vi "Auto-Pilot.vi"() -> ()   [LabVIEW 2017]
uses:
  <vilib>/Rock Robotics/WPI/DriverStation/WPI_DriverStationPositionInfo.ctl
  <vilib>/Rock Robotics/WPI/Utilities/WPI_GetSetVariantRefNum.vi
panel:
  out "Distance 6":dbl
  out "Distance 5":dbl
  out "Distance 2":dbl
  out "Distance":dbl
  out "substring":string
  out "Position":T1
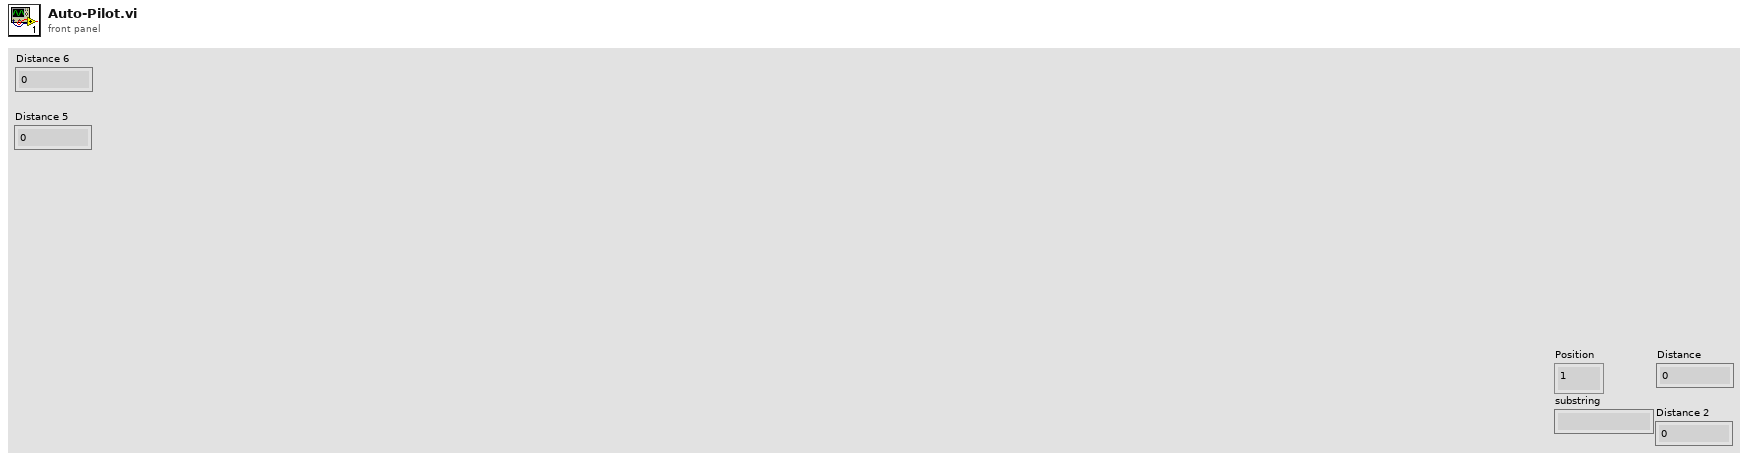
[diagram p1: front panel]
types:
  T1 = typedef "WPI_DriverStationPositionInfo.ctl" = enum16{"1", "2", "3"}
  T2 = typedef "WPI_EncoderDevRef.ctl" = cluster{"DevStatus":errorcluster, "EncoderIndex":T3, "CounterIndex":T4, "DistancePerCount":dbl, "Decoding Type":T5}
  T3 = typedef "FPGA_EncoderIdx.ctl" = enum8{"Enc 0", "Enc 1", "Enc 2", "Enc 3", "Enc 4", "Enc 5", "Enc 6", "Enc 7", "Invalid"}
  T4 = typedef "FPGA_CounterCtrSystemIndex.ctl" = enum8{"Ctr 0", "Ctr 1", "Ctr 2", "Ctr 3", "Ctr 4", "Ctr 5", "Ctr 6", "Ctr 7", "Invalid"}
  T5 = typedef "WPI_EncoderType.ctl" = enum16{"1x", "2x", "4x"}
  T6 = typedef "WPI_RobotDriveDevRef.ctl" = cluster{"DevStatus":errorcluster, "Motors[]":T7[], "Square Inputs":bool, "Max Output":dbl}
  T7 = typedef "WPI_MotorControlDeviceRef.ctl" = cluster{"DeviceStatus":errorcluster, "Type":T8, "PWM":cluster{"PWM Channel":T9, "DeadBand":T10}, "CAN":cluster{"Device Number":u8, "SetOutput VI Ref":variant, "GetOutput VI Ref":variant, "Enable VI Ref":variant, "Disable VI Ref":variant, "Data":variant}, "Invert":bool, "DIO PWM":cluster{"PWM \"Enable\" Channel":T9, "DIOChannel":T11, "PWM Rate":dbl}}
  T8 = typedef "WPI_MotorControlType.ctl" = enum16{"PWM", "CAN", "DIO PWM"}
  T9 = typedef "FPGA_DIOPWMChannel.ctl" = enum8{"PWM 0", "PWM 1", "PWM 2", "PWM 3", "PWM 4", "PWM 5", "PWM 6", "PWM 7", "PWM 8", "PWM 9", "PWM MXP 0", "PWM MXP 1", "PWM MXP 2", "PWM MXP 3", "PWM MXP 4", "PWM MXP 5", "PWM MXP 6", "PWM MXP 7", "PWM MXP 8", "PWM MXP 9", "Invalid"}
  T10 = typedef "WPI_PWMDeadband.ctl" = cluster{"Name":string, "maxPositivePwm":i32, "minPositivePwm":i32, "centerPwm":i32, "maxNegativePwm":i32, "minNegativePwm":i32, "angularRange":u16}
  T11 = typedef "FPGA_DIOChannel.ctl" = enum8{"DIO 0", "DIO 1", "DIO 2", "DIO 3", "DIO 4", "DIO 5", "DIO 6", "DIO 7", "DIO 8", "DIO 9", "DIO MXP 0", "DIO MXP 1", "DIO MXP 2", "DIO MXP 3", "DIO MXP 4", "DIO MXP 5", "DIO MXP 6", "DIO MXP 7", "DIO MXP 8", "DIO MXP 9", "DIO MXP 10", "DIO MXP 11", "DIO MXP 12", "DIO MXP 13", "DIO MXP 14", "DIO MXP 15", "SPI Port CS1", "SPI Port CS2", "SPI Port CS3", "SPI Port MISO", "SPI Port MOSI", "Invalid"}
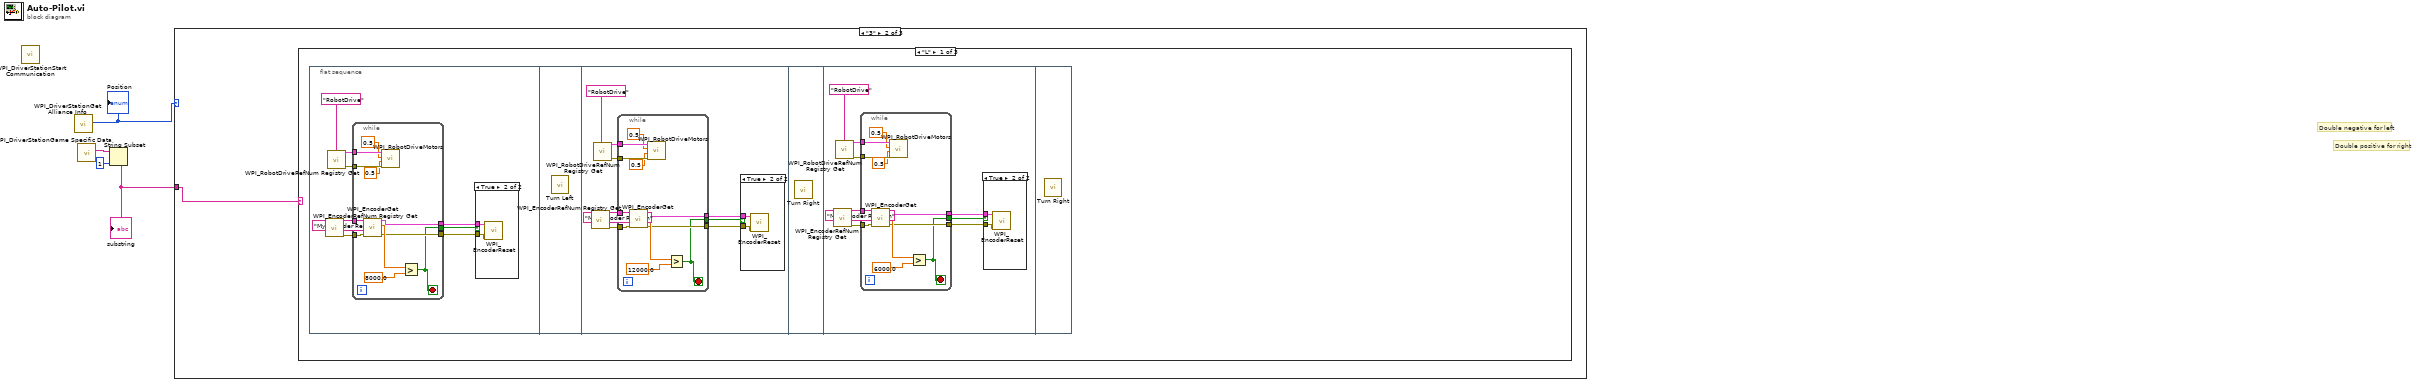
[diagram p0: block diagram]
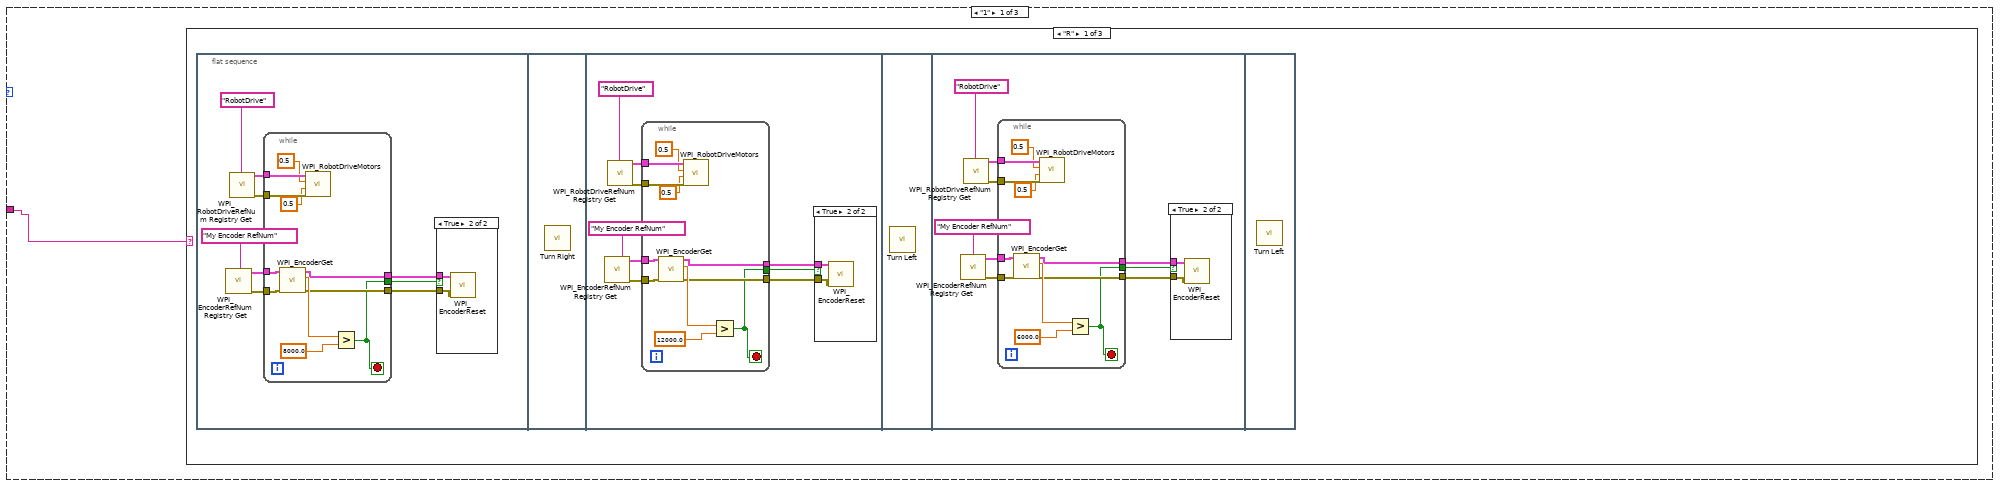
[diagram p2: hidden frame]
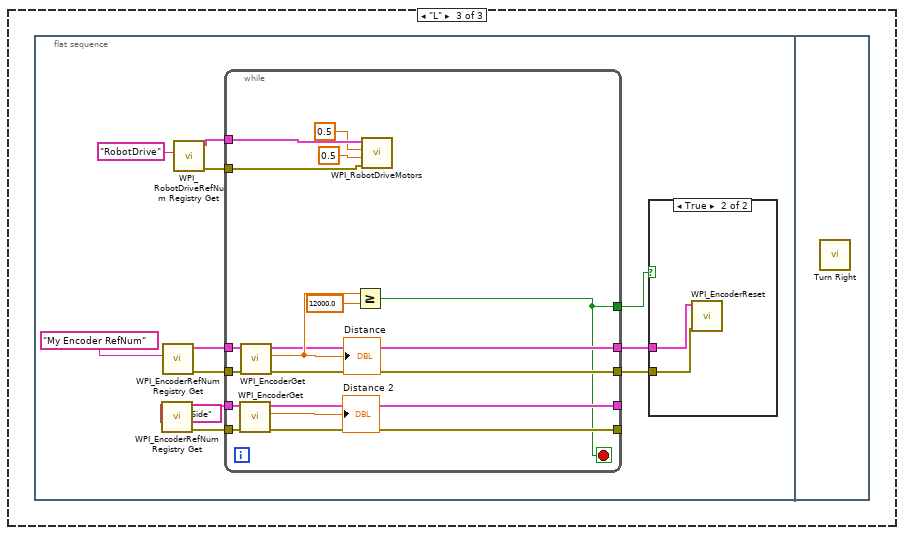
[diagram p7: hidden frame]
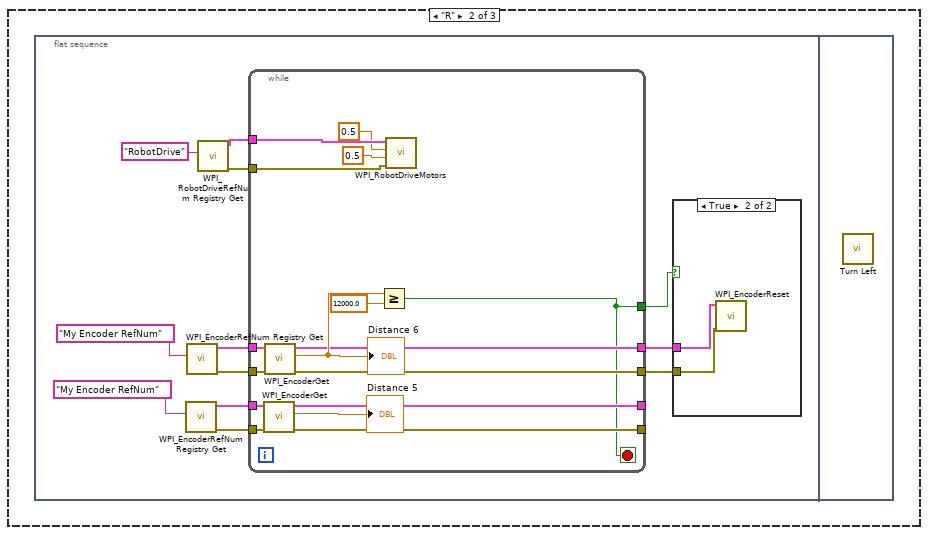
[diagram p12: hidden frame]
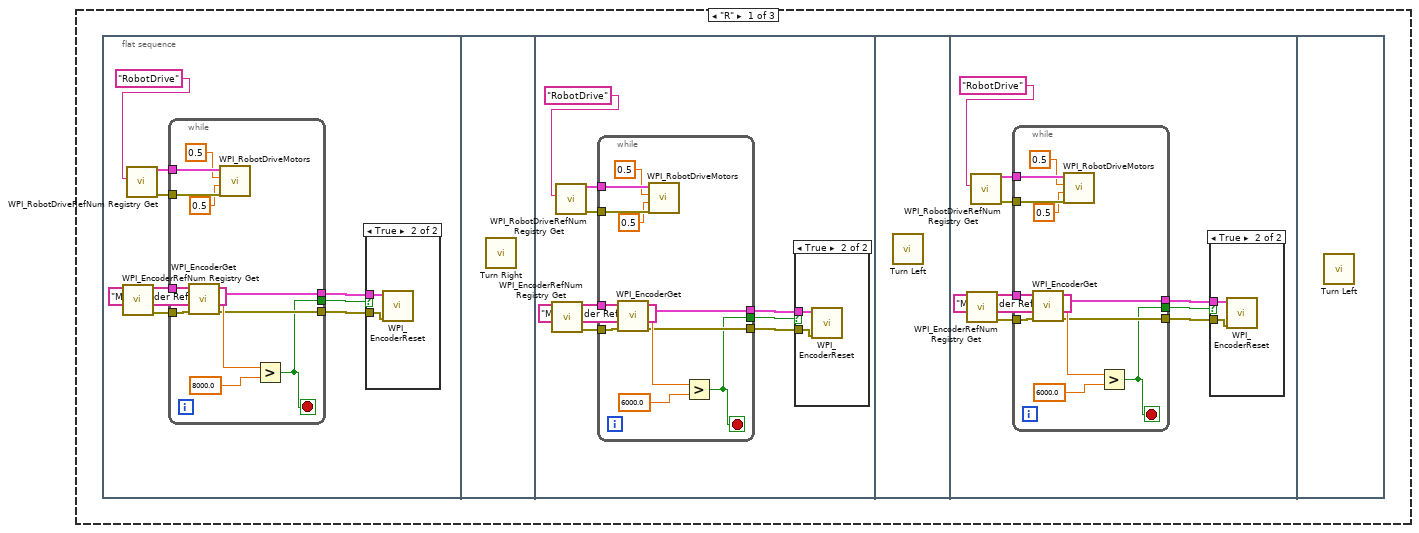
[diagram p16: hidden frame]
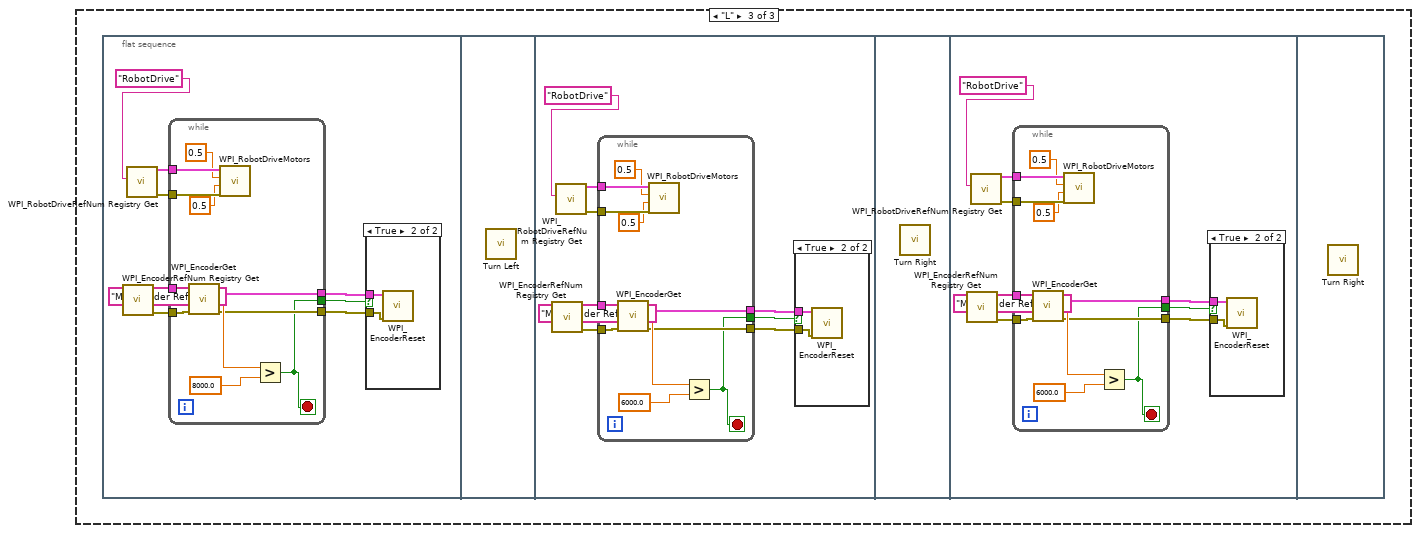
[diagram p20: hidden frame]
diagram:
  # "Double positive for right"
  # "Double negative for left"
  n1 = call <vilib>:"WPI_DriverStationStart Communication.vi"() -> ()  [unwired: 12 in]
  n2 = call <vilib>:"WPI_DriverStationGet Alliance Info.vi"() -> ("Position"=w2:T1)  [unwired: 6 in, 5 out]
  "Position" <- w2
  n3 = call <vilib>:"WPI_DriverStationGame Specific Data.vi"() -> ("Game Specific Data"=w4:string)  [unwired: 11 in]
  n4 = String Subset(string=w4, length (rest)=1 ("length (rest)")) -> (substring=w1:string)  [unwired: 1 in]
  "substring" <- w1
  n5 = case shown="\"3\"" w2 {
    tunnel: w1 -> [w5 w102 w199]
    frame "1" {
      n6 = case shown="\"R\"" w5 {
        frame "R" {
          n7 = flat-sequence {
            frame #0 {
              n8 = call <vilib>:"WPI_EncoderRefNum Registry Get.vi"("refnum name"="My Encoder RefNum") -> ("error out"=w10:errorcluster, "EncoderDevRef"=w11:T2)  [unwired: 9 in]
              n9 = call <vilib>:"WPI_RobotDriveRefNum Registry Get.vi"("refnum name"="RobotDrive") -> ("error out"=w13:errorcluster, "RobotDriveDevRef"=w14:T6)  [unwired: 9 in]
              n10 = while {
                tunnel: w14 -> [w27]
                tunnel: w13 -> [w26]
                tunnel: w11 -> [w23]
                tunnel: w10 -> [w22]
                tunnel: [w19] -> w9
                tunnel: [w18] -> w8
                tunnel: [w17] -> w7
                stop <- w17 stop-if-true
                n11 = call <vilib>:"WPI_EncoderGet.vi"("error in (no error)"=w22, "EncoderDevRef"=w23) -> ("error out"=w18:errorcluster, "Distance"=w21:dbl, "EncoderDevRef"=w19:T2)  [unwired: 4 in, 3 out]
                n12 = call <vilib>:"WPI_RobotDriveMotors.vi"("error in (no error)"=w26, "RightSpeed"=0.5, "LeftSpeed"=0.5, "RobotDriveDevRef"=w27) -> ()  [unwired: 5 in, 3 out]
                n13 = Greater?(x=w21, y=8000.0) -> (0:w17:bool)
              }
              n14 = case shown="True" w7 {
                tunnel: w9 -> [_ w16]
                tunnel: w8 -> [_ w15]
                frame False {
                }
                frame True {
                  n15 = call <vilib>:"WPI_EncoderReset.vi"("error in (no error)"=w15, "EncoderDevRef"=w16) -> ()  [unwired: 8 in, 2 out]
                }
              }
            }
            frame #1 {
              n16 = call "Turn Right.vi"() -> ()  [unwired: 12 in]
            }
            frame #2 {
              n17 = call <vilib>:"WPI_EncoderRefNum Registry Get.vi"("refnum name"="My Encoder RefNum") -> ("error out"=w33:errorcluster, "EncoderDevRef"=w32:T2)  [unwired: 9 in]
              n18 = call <vilib>:"WPI_RobotDriveRefNum Registry Get.vi"("refnum name"="RobotDrive") -> ("error out"=w30:errorcluster, "RobotDriveDevRef"=w29:T6)  [unwired: 9 in]
              n19 = while {
                tunnel: w29 -> [w49]
                tunnel: w30 -> [w48]
                tunnel: w32 -> [w45]
                tunnel: w33 -> [w44]
                tunnel: [w41] -> w34
                tunnel: [w40] -> w35
                tunnel: [w39] -> w36
                stop <- w39 stop-if-true
                n20 = call <vilib>:"WPI_EncoderGet.vi"("error in (no error)"=w44, "EncoderDevRef"=w45) -> ("error out"=w40:errorcluster, "Distance"=w43:dbl, "EncoderDevRef"=w41:T2)  [unwired: 4 in, 3 out]
                n21 = call <vilib>:"WPI_RobotDriveMotors.vi"("error in (no error)"=w48, "RightSpeed"=0.5, "LeftSpeed"=0.5, "RobotDriveDevRef"=w49) -> ()  [unwired: 5 in, 3 out]
                n22 = Greater?(x=w43, y=12000.0) -> (0:w39:bool)
              }
              n23 = case shown="True" w36 {
                tunnel: w34 -> [_ w38]
                tunnel: w35 -> [_ w37]
                frame False {
                }
                frame True {
                  n24 = call <vilib>:"WPI_EncoderReset.vi"("error in (no error)"=w37, "EncoderDevRef"=w38) -> ()  [unwired: 8 in, 2 out]
                }
              }
            }
            frame #3 {
              n25 = call "Turn Left.vi"() -> ()  [unwired: 12 in]
            }
            frame #4 {
              n26 = call <vilib>:"WPI_EncoderRefNum Registry Get.vi"("refnum name"="My Encoder RefNum") -> ("error out"=w54:errorcluster, "EncoderDevRef"=w55:T2)  [unwired: 9 in]
              n27 = call <vilib>:"WPI_RobotDriveRefNum Registry Get.vi"("refnum name"="RobotDrive") -> ("error out"=w57:errorcluster, "RobotDriveDevRef"=w58:T6)  [unwired: 9 in]
              n28 = while {
                tunnel: w58 -> [w71]
                tunnel: w57 -> [w70]
                tunnel: w55 -> [w67]
                tunnel: w54 -> [w66]
                tunnel: [w63] -> w53
                tunnel: [w62] -> w52
                tunnel: [w61] -> w51
                stop <- w61 stop-if-true
                n29 = call <vilib>:"WPI_EncoderGet.vi"("error in (no error)"=w66, "EncoderDevRef"=w67) -> ("error out"=w62:errorcluster, "Distance"=w65:dbl, "EncoderDevRef"=w63:T2)  [unwired: 4 in, 3 out]
                n30 = call <vilib>:"WPI_RobotDriveMotors.vi"("error in (no error)"=w70, "RightSpeed"=0.5, "LeftSpeed"=0.5, "RobotDriveDevRef"=w71) -> ()  [unwired: 5 in, 3 out]
                n31 = Greater?(x=w65, y=6000.0) -> (0:w61:bool)
              }
              n32 = case shown="True" w51 {
                tunnel: w53 -> [_ w60]
                tunnel: w52 -> [_ w59]
                frame False {
                }
                frame True {
                  n33 = call <vilib>:"WPI_EncoderReset.vi"("error in (no error)"=w59, "EncoderDevRef"=w60) -> ()  [unwired: 8 in, 2 out]
                }
              }
            }
            frame #5 {
              n34 = call "Turn Left.vi"() -> ()  [unwired: 12 in]
            }
          }
        }
        frame Default {
        }
        frame "L" {
          n35 = flat-sequence {
            frame #0 {
              n36 = call <vilib>:"WPI_EncoderRefNum Registry Get.vi"("refnum name"="Right Side") -> ("error out"=w81:errorcluster, "EncoderDevRef"=w80:T2)  [unwired: 9 in]
              n37 = call <vilib>:"WPI_EncoderRefNum Registry Get.vi"("refnum name"="My Encoder RefNum") -> ("error out"=w82:errorcluster, "EncoderDevRef"=w83:T2)  [unwired: 9 in]
              n38 = call <vilib>:"WPI_RobotDriveRefNum Registry Get.vi"("refnum name"="RobotDrive") -> ("error out"=w72:errorcluster, "RobotDriveDevRef"=w73:T6)  [unwired: 9 in]
              n39 = while {
                tunnel: w83 -> [w101]
                tunnel: w82 -> [w100]
                tunnel: w80 -> [w97]
                tunnel: w81 -> [w98]
                tunnel: [w94] -> w76
                tunnel: [w93] -> w75
                tunnel: [w92] -> _
                tunnel: [w91] -> _
                tunnel: [w90] -> w77
                tunnel: w73 -> [w89]
                tunnel: w72 -> [w88]
                stop <- w90 stop-if-true
                n40 = call <vilib>:"WPI_EncoderGet.vi"("error in (no error)"=w98, "EncoderDevRef"=w97) -> ("error out"=w91:errorcluster, "Distance"=→"Distance 2":dbl, "EncoderDevRef"=w92:T2)  [unwired: 4 in, 3 out]
                n41 = call <vilib>:"WPI_EncoderGet.vi"("error in (no error)"=w100, "EncoderDevRef"=w101) -> ("error out"=w93:errorcluster, "Distance"=w96:dbl, "EncoderDevRef"=w94:T2)  [unwired: 4 in, 3 out]
                "Distance" <- w96
                n42 = Greater Or Equal?(x=w96, y=12000.0) -> (x >= y?=w90:bool)
                n43 = call <vilib>:"WPI_RobotDriveMotors.vi"("error in (no error)"=w88, "RightSpeed"=0.5, "LeftSpeed"=0.5, "RobotDriveDevRef"=w89) -> ()  [unwired: 5 in, 3 out]
              }
              n44 = case shown="True" w77 {
                tunnel: w76 -> [_ w85]
                tunnel: w75 -> [_ w84]
                frame False {
                }
                frame True {
                  n45 = call <vilib>:"WPI_EncoderReset.vi"("error in (no error)"=w84, "EncoderDevRef"=w85) -> ()  [unwired: 8 in, 2 out]
                }
              }
            }
            frame #1 {
              n46 = call "Turn Right.vi"() -> ()  [unwired: 12 in]
            }
          }
        }
      }
    }
    frame "3" {
      n47 = case shown="\"L\"" w102 {
        frame "L" {
          n48 = flat-sequence {
            frame #0 {
              n49 = call <vilib>:"WPI_EncoderRefNum Registry Get.vi"("refnum name"="My Encoder RefNum") -> ("error out"=w107:errorcluster, "EncoderDevRef"=w108:T2)  [unwired: 9 in]
              n50 = call <vilib>:"WPI_RobotDriveRefNum Registry Get.vi"("refnum name"="RobotDrive") -> ("error out"=w110:errorcluster, "RobotDriveDevRef"=w111:T6)  [unwired: 9 in]
              n51 = while {
                tunnel: w111 -> [w124]
                tunnel: w110 -> [w123]
                tunnel: w108 -> [w120]
                tunnel: w107 -> [w119]
                tunnel: [w116] -> w106
                tunnel: [w115] -> w105
                tunnel: [w114] -> w104
                stop <- w114 stop-if-true
                n52 = call <vilib>:"WPI_EncoderGet.vi"("error in (no error)"=w119, "EncoderDevRef"=w120) -> ("error out"=w115:errorcluster, "Distance"=w118:dbl, "EncoderDevRef"=w116:T2)  [unwired: 4 in, 3 out]
                n53 = call <vilib>:"WPI_RobotDriveMotors.vi"("error in (no error)"=w123, "RightSpeed"=0.5, "LeftSpeed"=0.5, "RobotDriveDevRef"=w124) -> ()  [unwired: 5 in, 3 out]
                n54 = Greater?(x=w118, y=8000.0) -> (0:w114:bool)
              }
              n55 = case shown="True" w104 {
                tunnel: w106 -> [_ w113]
                tunnel: w105 -> [_ w112]
                frame False {
                }
                frame True {
                  n56 = call <vilib>:"WPI_EncoderReset.vi"("error in (no error)"=w112, "EncoderDevRef"=w113) -> ()  [unwired: 8 in, 2 out]
                }
              }
            }
            frame #1 {
              n57 = call "Turn Left.vi"() -> ()  [unwired: 12 in]
            }
            frame #2 {
              n58 = call <vilib>:"WPI_EncoderRefNum Registry Get.vi"("refnum name"="My Encoder RefNum") -> ("error out"=w130:errorcluster, "EncoderDevRef"=w129:T2)  [unwired: 9 in]
              n59 = call <vilib>:"WPI_RobotDriveRefNum Registry Get.vi"("refnum name"="RobotDrive") -> ("error out"=w127:errorcluster, "RobotDriveDevRef"=w126:T6)  [unwired: 9 in]
              n60 = while {
                tunnel: w126 -> [w146]
                tunnel: w127 -> [w145]
                tunnel: w129 -> [w142]
                tunnel: w130 -> [w141]
                tunnel: [w138] -> w131
                tunnel: [w137] -> w132
                tunnel: [w136] -> w133
                stop <- w136 stop-if-true
                n61 = call <vilib>:"WPI_EncoderGet.vi"("error in (no error)"=w141, "EncoderDevRef"=w142) -> ("error out"=w137:errorcluster, "Distance"=w140:dbl, "EncoderDevRef"=w138:T2)  [unwired: 4 in, 3 out]
                n62 = call <vilib>:"WPI_RobotDriveMotors.vi"("error in (no error)"=w145, "RightSpeed"=0.5, "LeftSpeed"=0.5, "RobotDriveDevRef"=w146) -> ()  [unwired: 5 in, 3 out]
                n63 = Greater?(x=w140, y=12000.0) -> (0:w136:bool)
              }
              n64 = case shown="True" w133 {
                tunnel: w131 -> [_ w135]
                tunnel: w132 -> [_ w134]
                frame False {
                }
                frame True {
                  n65 = call <vilib>:"WPI_EncoderReset.vi"("error in (no error)"=w134, "EncoderDevRef"=w135) -> ()  [unwired: 8 in, 2 out]
                }
              }
            }
            frame #3 {
              n66 = call "Turn Right.vi"() -> ()  [unwired: 12 in]
            }
            frame #4 {
              n67 = call <vilib>:"WPI_EncoderRefNum Registry Get.vi"("refnum name"="My Encoder RefNum") -> ("error out"=w151:errorcluster, "EncoderDevRef"=w152:T2)  [unwired: 9 in]
              n68 = call <vilib>:"WPI_RobotDriveRefNum Registry Get.vi"("refnum name"="RobotDrive") -> ("error out"=w154:errorcluster, "RobotDriveDevRef"=w155:T6)  [unwired: 9 in]
              n69 = while {
                tunnel: w155 -> [w168]
                tunnel: w154 -> [w167]
                tunnel: w152 -> [w164]
                tunnel: w151 -> [w163]
                tunnel: [w160] -> w150
                tunnel: [w159] -> w149
                tunnel: [w158] -> w148
                stop <- w158 stop-if-true
                n70 = call <vilib>:"WPI_EncoderGet.vi"("error in (no error)"=w163, "EncoderDevRef"=w164) -> ("error out"=w159:errorcluster, "Distance"=w162:dbl, "EncoderDevRef"=w160:T2)  [unwired: 4 in, 3 out]
                n71 = call <vilib>:"WPI_RobotDriveMotors.vi"("error in (no error)"=w167, "RightSpeed"=0.5, "LeftSpeed"=0.5, "RobotDriveDevRef"=w168) -> ()  [unwired: 5 in, 3 out]
                n72 = Greater?(x=w162, y=6000.0) -> (0:w158:bool)
              }
              n73 = case shown="True" w148 {
                tunnel: w150 -> [_ w157]
                tunnel: w149 -> [_ w156]
                frame False {
                }
                frame True {
                  n74 = call <vilib>:"WPI_EncoderReset.vi"("error in (no error)"=w156, "EncoderDevRef"=w157) -> ()  [unwired: 8 in, 2 out]
                }
              }
            }
            frame #5 {
              n75 = call "Turn Right.vi"() -> ()  [unwired: 12 in]
            }
          }
        }
        frame "R" {
          n76 = flat-sequence {
            frame #0 {
              n77 = call <vilib>:"WPI_EncoderRefNum Registry Get.vi"("refnum name"="My Encoder RefNum") -> ("error out"=w178:errorcluster, "EncoderDevRef"=w177:T2)  [unwired: 9 in]
              n78 = call <vilib>:"WPI_EncoderRefNum Registry Get.vi"("refnum name"="My Encoder RefNum") -> ("error out"=w179:errorcluster, "EncoderDevRef"=w180:T2)  [unwired: 9 in]
              n79 = call <vilib>:"WPI_RobotDriveRefNum Registry Get.vi"("refnum name"="RobotDrive") -> ("error out"=w169:errorcluster, "RobotDriveDevRef"=w170:T6)  [unwired: 9 in]
              n80 = while {
                tunnel: w180 -> [w198]
                tunnel: w179 -> [w197]
                tunnel: w177 -> [w194]
                tunnel: w178 -> [w195]
                tunnel: [w191] -> w173
                tunnel: [w190] -> w172
                tunnel: [w189] -> _
                tunnel: [w188] -> _
                tunnel: [w187] -> w174
                tunnel: w170 -> [w186]
                tunnel: w169 -> [w185]
                stop <- w187 stop-if-true
                n81 = call <vilib>:"WPI_EncoderGet.vi"("error in (no error)"=w195, "EncoderDevRef"=w194) -> ("error out"=w188:errorcluster, "Distance"=→"Distance 5":dbl, "EncoderDevRef"=w189:T2)  [unwired: 4 in, 3 out]
                n82 = call <vilib>:"WPI_EncoderGet.vi"("error in (no error)"=w197, "EncoderDevRef"=w198) -> ("error out"=w190:errorcluster, "Distance"=w193:dbl, "EncoderDevRef"=w191:T2)  [unwired: 4 in, 3 out]
                "Distance 6" <- w193
                n83 = Greater Or Equal?(x=w193, y=12000.0) -> (x >= y?=w187:bool)
                n84 = call <vilib>:"WPI_RobotDriveMotors.vi"("error in (no error)"=w185, "RightSpeed"=0.5, "LeftSpeed"=0.5, "RobotDriveDevRef"=w186) -> ()  [unwired: 5 in, 3 out]
              }
              n85 = case shown="True" w174 {
                tunnel: w173 -> [_ w182]
                tunnel: w172 -> [_ w181]
                frame False {
                }
                frame True {
                  n86 = call <vilib>:"WPI_EncoderReset.vi"("error in (no error)"=w181, "EncoderDevRef"=w182) -> ()  [unwired: 8 in, 2 out]
                }
              }
            }
            frame #1 {
              n87 = call "Turn Left.vi"() -> ()  [unwired: 12 in]
            }
          }
        }
        frame Default {
        }
      }
    }
    frame "2" {
      n88 = case shown="Default" w199 {
        frame "R" {
          n89 = flat-sequence {
            frame #0 {
              n90 = call <vilib>:"WPI_EncoderRefNum Registry Get.vi"("refnum name"="My Encoder RefNum") -> ("error out"=w205:errorcluster, "EncoderDevRef"=w204:T2)  [unwired: 9 in]
              n91 = call <vilib>:"WPI_RobotDriveRefNum Registry Get.vi"("refnum name"="RobotDrive") -> ("error out"=w203:errorcluster, "RobotDriveDevRef"=w202:T6)  [unwired: 9 in]
              n92 = while {
                tunnel: w202 -> [w221]
                tunnel: w203 -> [w220]
                tunnel: w204 -> [w217]
                tunnel: w205 -> [w216]
                tunnel: [w213] -> w206
                tunnel: [w212] -> w207
                tunnel: [w211] -> w208
                stop <- w211 stop-if-true
                n93 = call <vilib>:"WPI_EncoderGet.vi"("error in (no error)"=w216, "EncoderDevRef"=w217) -> ("error out"=w212:errorcluster, "Distance"=w215:dbl, "EncoderDevRef"=w213:T2)  [unwired: 4 in, 3 out]
                n94 = call <vilib>:"WPI_RobotDriveMotors.vi"("error in (no error)"=w220, "RightSpeed"=0.5, "LeftSpeed"=0.5, "RobotDriveDevRef"=w221) -> ()  [unwired: 5 in, 3 out]
                n95 = Greater?(x=w215, y=8000.0) -> (0:w211:bool)
              }
              n96 = case shown="True" w208 {
                tunnel: w206 -> [_ w210]
                tunnel: w207 -> [_ w209]
                frame False {
                }
                frame True {
                  n97 = call <vilib>:"WPI_EncoderReset.vi"("error in (no error)"=w209, "EncoderDevRef"=w210) -> ()  [unwired: 8 in, 2 out]
                }
              }
            }
            frame #1 {
              n98 = call "Turn Right.vi"() -> ()  [unwired: 12 in]
            }
            frame #2 {
              n99 = call <vilib>:"WPI_EncoderRefNum Registry Get.vi"("refnum name"="My Encoder RefNum") -> ("error out"=w226:errorcluster, "EncoderDevRef"=w227:T2)  [unwired: 9 in]
              n100 = call <vilib>:"WPI_RobotDriveRefNum Registry Get.vi"("refnum name"="RobotDrive") -> ("error out"=w228:errorcluster, "RobotDriveDevRef"=w229:T6)  [unwired: 9 in]
              n101 = while {
                tunnel: w229 -> [w243]
                tunnel: w228 -> [w242]
                tunnel: w227 -> [w239]
                tunnel: w226 -> [w238]
                tunnel: [w235] -> w225
                tunnel: [w234] -> w224
                tunnel: [w233] -> w223
                stop <- w233 stop-if-true
                n102 = call <vilib>:"WPI_EncoderGet.vi"("error in (no error)"=w238, "EncoderDevRef"=w239) -> ("error out"=w234:errorcluster, "Distance"=w237:dbl, "EncoderDevRef"=w235:T2)  [unwired: 4 in, 3 out]
                n103 = call <vilib>:"WPI_RobotDriveMotors.vi"("error in (no error)"=w242, "RightSpeed"=0.5, "LeftSpeed"=0.5, "RobotDriveDevRef"=w243) -> ()  [unwired: 5 in, 3 out]
                n104 = Greater?(x=w237, y=6000.0) -> (0:w233:bool)
              }
              n105 = case shown="True" w223 {
                tunnel: w225 -> [_ w232]
                tunnel: w224 -> [_ w231]
                frame False {
                }
                frame True {
                  n106 = call <vilib>:"WPI_EncoderReset.vi"("error in (no error)"=w231, "EncoderDevRef"=w232) -> ()  [unwired: 8 in, 2 out]
                }
              }
            }
            frame #3 {
              n107 = call "Turn Left.vi"() -> ()  [unwired: 12 in]
            }
            frame #4 {
              n108 = call <vilib>:"WPI_EncoderRefNum Registry Get.vi"("refnum name"="My Encoder RefNum") -> ("error out"=w249:errorcluster, "EncoderDevRef"=w248:T2)  [unwired: 9 in]
              n109 = call <vilib>:"WPI_RobotDriveRefNum Registry Get.vi"("refnum name"="RobotDrive") -> ("error out"=w247:errorcluster, "RobotDriveDevRef"=w246:T6)  [unwired: 9 in]
              n110 = while {
                tunnel: w246 -> [w265]
                tunnel: w247 -> [w264]
                tunnel: w248 -> [w261]
                tunnel: w249 -> [w260]
                tunnel: [w257] -> w250
                tunnel: [w256] -> w251
                tunnel: [w255] -> w252
                stop <- w255 stop-if-true
                n111 = call <vilib>:"WPI_EncoderGet.vi"("error in (no error)"=w260, "EncoderDevRef"=w261) -> ("error out"=w256:errorcluster, "Distance"=w259:dbl, "EncoderDevRef"=w257:T2)  [unwired: 4 in, 3 out]
                n112 = call <vilib>:"WPI_RobotDriveMotors.vi"("error in (no error)"=w264, "RightSpeed"=0.5, "LeftSpeed"=0.5, "RobotDriveDevRef"=w265) -> ()  [unwired: 5 in, 3 out]
                n113 = Greater?(x=w259, y=6000.0) -> (0:w255:bool)
              }
              n114 = case shown="True" w252 {
                tunnel: w250 -> [_ w254]
                tunnel: w251 -> [_ w253]
                frame False {
                }
                frame True {
                  n115 = call <vilib>:"WPI_EncoderReset.vi"("error in (no error)"=w253, "EncoderDevRef"=w254) -> ()  [unwired: 8 in, 2 out]
                }
              }
            }
            frame #5 {
              n116 = call "Turn Left.vi"() -> ()  [unwired: 12 in]
            }
          }
        }
        frame Default {
        }
        frame "L" {
          n117 = flat-sequence {
            frame #0 {
              n118 = call <vilib>:"WPI_EncoderRefNum Registry Get.vi"("refnum name"="My Encoder RefNum") -> ("error out"=w271:errorcluster, "EncoderDevRef"=w270:T2)  [unwired: 9 in]
              n119 = call <vilib>:"WPI_RobotDriveRefNum Registry Get.vi"("refnum name"="RobotDrive") -> ("error out"=w269:errorcluster, "RobotDriveDevRef"=w268:T6)  [unwired: 9 in]
              n120 = while {
                tunnel: w268 -> [w287]
                tunnel: w269 -> [w286]
                tunnel: w270 -> [w283]
                tunnel: w271 -> [w282]
                tunnel: [w279] -> w272
                tunnel: [w278] -> w273
                tunnel: [w277] -> w274
                stop <- w277 stop-if-true
                n121 = call <vilib>:"WPI_EncoderGet.vi"("error in (no error)"=w282, "EncoderDevRef"=w283) -> ("error out"=w278:errorcluster, "Distance"=w281:dbl, "EncoderDevRef"=w279:T2)  [unwired: 4 in, 3 out]
                n122 = call <vilib>:"WPI_RobotDriveMotors.vi"("error in (no error)"=w286, "RightSpeed"=0.5, "LeftSpeed"=0.5, "RobotDriveDevRef"=w287) -> ()  [unwired: 5 in, 3 out]
                n123 = Greater?(x=w281, y=8000.0) -> (0:w277:bool)
              }
              n124 = case shown="True" w274 {
                tunnel: w272 -> [_ w276]
                tunnel: w273 -> [_ w275]
                frame False {
                }
                frame True {
                  n125 = call <vilib>:"WPI_EncoderReset.vi"("error in (no error)"=w275, "EncoderDevRef"=w276) -> ()  [unwired: 8 in, 2 out]
                }
              }
            }
            frame #1 {
              n126 = call "Turn Left.vi"() -> ()  [unwired: 12 in]
            }
            frame #2 {
              n127 = call <vilib>:"WPI_EncoderRefNum Registry Get.vi"("refnum name"="My Encoder RefNum") -> ("error out"=w292:errorcluster, "EncoderDevRef"=w293:T2)  [unwired: 9 in]
              n128 = call <vilib>:"WPI_RobotDriveRefNum Registry Get.vi"("refnum name"="RobotDrive") -> ("error out"=w294:errorcluster, "RobotDriveDevRef"=w295:T6)  [unwired: 9 in]
              n129 = while {
                tunnel: w295 -> [w309]
                tunnel: w294 -> [w308]
                tunnel: w293 -> [w305]
                tunnel: w292 -> [w304]
                tunnel: [w301] -> w291
                tunnel: [w300] -> w290
                tunnel: [w299] -> w289
                stop <- w299 stop-if-true
                n130 = call <vilib>:"WPI_EncoderGet.vi"("error in (no error)"=w304, "EncoderDevRef"=w305) -> ("error out"=w300:errorcluster, "Distance"=w303:dbl, "EncoderDevRef"=w301:T2)  [unwired: 4 in, 3 out]
                n131 = call <vilib>:"WPI_RobotDriveMotors.vi"("error in (no error)"=w308, "RightSpeed"=0.5, "LeftSpeed"=0.5, "RobotDriveDevRef"=w309) -> ()  [unwired: 5 in, 3 out]
                n132 = Greater?(x=w303, y=6000.0) -> (0:w299:bool)
              }
              n133 = case shown="True" w289 {
                tunnel: w291 -> [_ w298]
                tunnel: w290 -> [_ w297]
                frame False {
                }
                frame True {
                  n134 = call <vilib>:"WPI_EncoderReset.vi"("error in (no error)"=w297, "EncoderDevRef"=w298) -> ()  [unwired: 8 in, 2 out]
                }
              }
            }
            frame #3 {
              n135 = call "Turn Right.vi"() -> ()  [unwired: 12 in]
            }
            frame #4 {
              n136 = call <vilib>:"WPI_EncoderRefNum Registry Get.vi"("refnum name"="My Encoder RefNum") -> ("error out"=w315:errorcluster, "EncoderDevRef"=w314:T2)  [unwired: 9 in]
              n137 = call <vilib>:"WPI_RobotDriveRefNum Registry Get.vi"("refnum name"="RobotDrive") -> ("error out"=w313:errorcluster, "RobotDriveDevRef"=w312:T6)  [unwired: 9 in]
              n138 = while {
                tunnel: w312 -> [w331]
                tunnel: w313 -> [w330]
                tunnel: w314 -> [w327]
                tunnel: w315 -> [w326]
                tunnel: [w323] -> w316
                tunnel: [w322] -> w317
                tunnel: [w321] -> w318
                stop <- w321 stop-if-true
                n139 = call <vilib>:"WPI_EncoderGet.vi"("error in (no error)"=w326, "EncoderDevRef"=w327) -> ("error out"=w322:errorcluster, "Distance"=w325:dbl, "EncoderDevRef"=w323:T2)  [unwired: 4 in, 3 out]
                n140 = call <vilib>:"WPI_RobotDriveMotors.vi"("error in (no error)"=w330, "RightSpeed"=0.5, "LeftSpeed"=0.5, "RobotDriveDevRef"=w331) -> ()  [unwired: 5 in, 3 out]
                n141 = Greater?(x=w325, y=6000.0) -> (0:w321:bool)
              }
              n142 = case shown="True" w318 {
                tunnel: w316 -> [_ w320]
                tunnel: w317 -> [_ w319]
                frame False {
                }
                frame True {
                  n143 = call <vilib>:"WPI_EncoderReset.vi"("error in (no error)"=w319, "EncoderDevRef"=w320) -> ()  [unwired: 8 in, 2 out]
                }
              }
            }
            frame #5 {
              n144 = call "Turn Right.vi"() -> ()  [unwired: 12 in]
            }
          }
        }
      }
    }
  }
